vi "identify.vi"(8 "error in (no error)":errorcluster, 11 "plugin_interface in":refnum<class "odbc_driver_postgres_v13.0.2.lvclass">) -> (0 "error out":errorcluster, 2 "identifier":string, 3 "plugin_interface out":refnum<class "odbc_driver_postgres_v13.0.2.lvclass">)   [LabVIEW 2015, in "lv-example-postgres-post-installer.lvlib" / "odbc_driver_postgres_v13.0.2.lvclass"]
uses:
  odbc_driver_postgres_v13.0.2.lvclass
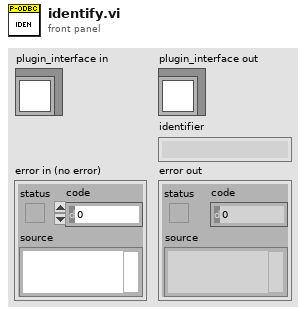
[diagram p1: front panel]
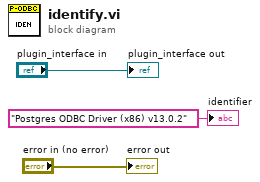
[diagram p0: block diagram]
diagram:
  "error out" <- "error in (no error)"
  "plugin_interface out" <- "plugin_interface in"
  "identifier" <- "Postgres ODBC Driver (x86) v13.0.2" ("identifier")
